vi "PhotonPoseEstimator_lowestAmbiguityStrategy.vi"(10 "CameraResult":T11, 11 "data value reference":T1) -> (1 "Pos Found":bool, 3 "PhotonEstimatedRobotPose":T2={"EstimatedPose"={"Translation3d"={"X"=0.0, "Y"=0.0, "Z"=0.0}, "Rotation3d"={"Q_quaternion"={"R"=1.0, "V"=[0.0, 0.0, 0.0]}}}, "TimeStamp_Seconds"=0.0, "targetsUsed"=[], "Strategy"=enum."LOWEST_AMBIGUITY"} {"targetsUsed"."AltCameraToTarget"."TRANSLATION3D"."Z" format="%14.3f"; "targetsUsed"."AltCameraToTarget"."TRANSLATION3D"."Y" format="%14.3f"; "targetsUsed"."AltCameraToTarget"."TRANSLATION3D"."X" format="%14.3f"; "targetsUsed"."BestCameraToTarget"."TRANSLATION3D"."Z" format="%14.3f"; "targetsUsed"."BestCameraToTarget"."TRANSLATION3D"."Y" format="%14.3f"; "targetsUsed"."BestCameraToTarget"."TRANSLATION3D"."X" format="%14.3f"; "EstimatedPose"."Translation3d"."Z" format="%14.3f"; "EstimatedPose"."Translation3d"."Y" format="%14.3f"; "EstimatedPose"."Translation3d"."X" format="%14.3f"})   [LabVIEW 2019, in "PhotonVisionLib.lvlib"]
doc: "This is an internal function. Use Update or Update_Pipeline instead of this function.\n\nDetermine the best target based the lowest ambiguity."
uses:
  PhotonVisionLib.lvlib
  TypeDef/TargetCornerType.ctl
  <vilib>/Rock Robotics/WPI/ThirdParty/JAS_Junk/TrajLib/TypeDef/TRANSLATION3D.ctl
  <vilib>/Rock Robotics/WPI/ThirdParty/JAS_Junk/TrajLib/Trajectory_Library.lvlib
  <vilib>/Rock Robotics/WPI/ThirdParty/JAS_Junk/TrajLib/TypeDef/QUATERNION.ctl
  <vilib>/Rock Robotics/WPI/ThirdParty/JAS_Junk/TrajLib/TypeDef/ROTATION3D.ctl
  <vilib>/Rock Robotics/WPI/ThirdParty/JAS_Junk/TrajLib/TypeDef/TRANSFORM3D.ctl
  TypeDef/PhotonTrackedTargetType.ctl
  Enum/PhotonPoseStrategy_ENUM.ctl
  <vilib>/Rock Robotics/WPI/ThirdParty/JAS_Junk/TrajLib/TypeDef/POSE3D.ctl
  TypeDef/PhotonEstimatedRobotPoseType.ctl
  TypeDef/PhotonPipelineResultType.ctl
  <vilib>/Rock Robotics/WPI/ThirdParty/JAS_Junk/TrajLib/TypeDef/AprilTag.ctl
  <vilib>/Rock Robotics/WPI/ThirdParty/JAS_Junk/TrajLib/Enum/AprilTagFieldLayoutOrignPosition_ENUM.ctl
  <vilib>/Rock Robotics/WPI/ThirdParty/JAS_Junk/TrajLib/TypeDef/AprilTagFieldLayout.ctl
  TypeDef/PhotonPoseEstimatorType.ctl
  TypeDef/PhotonPNPResultType.ctl
  TypeDef/PhotonMultiTargetPNPResultType.ctl
  TypeDef/PhotonTargetModel.ctl
  Ref/PhotonPipelineResult_REF.ctl
  Ref/PhotonPoseEstimator_REF.ctl
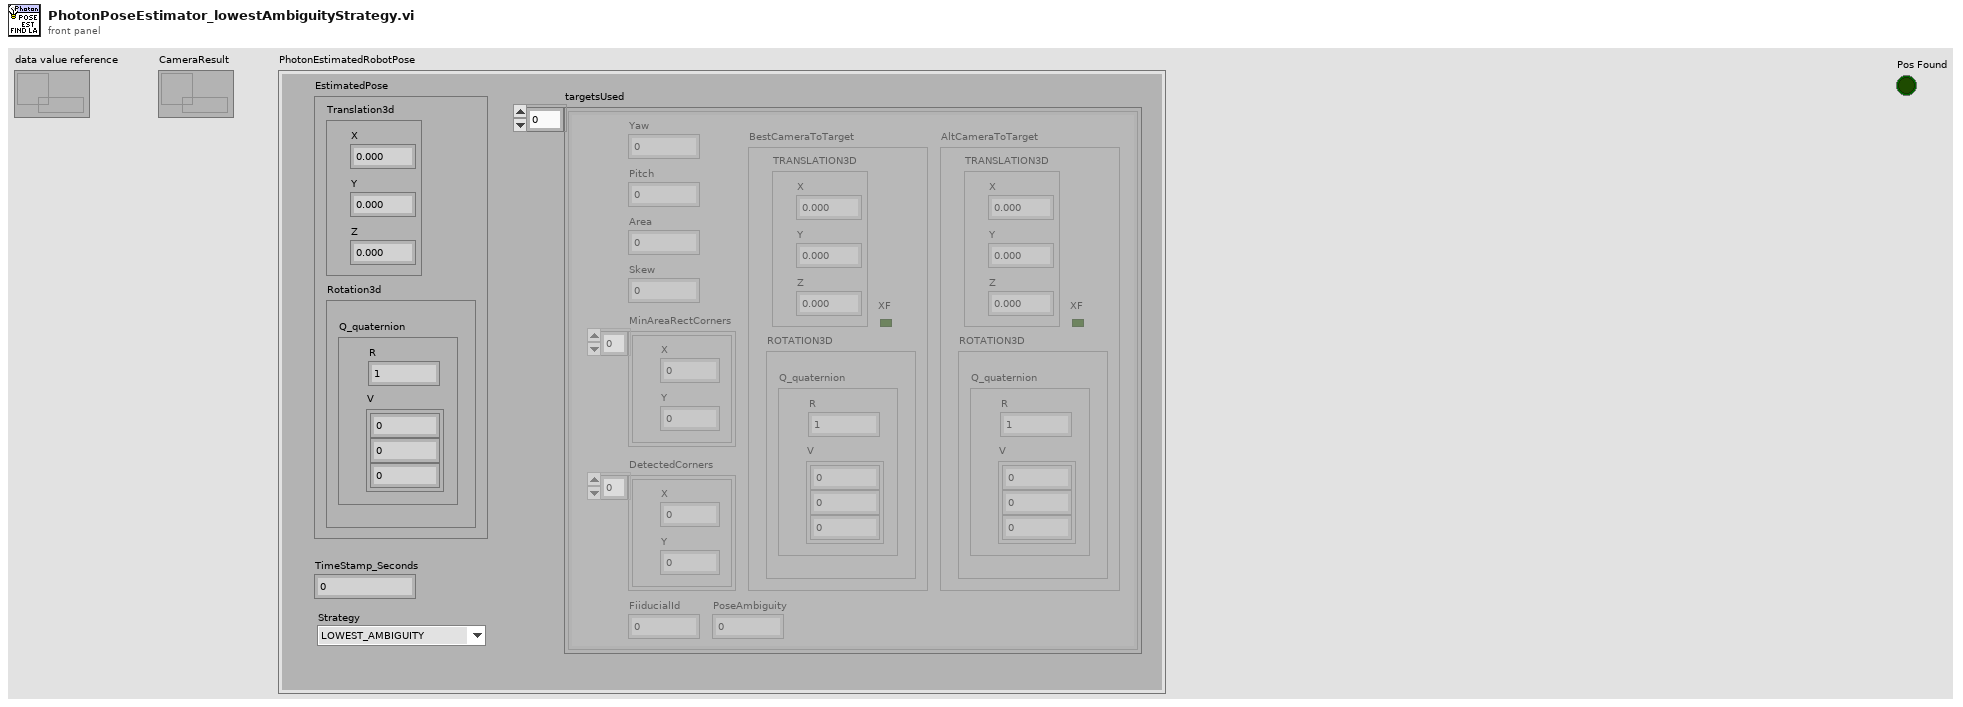
[diagram p1: front panel]
types:
  T1 = typedef "PhotonVisionLib.lvlib/PhotonPoseEstimator_REF.ctl" = refnum<data-value>
  T2 = typedef "PhotonVisionLib.lvlib/PhotonEstimatedRobotPoseType.ctl" = cluster{"EstimatedPose":T3, "TimeStamp_Seconds":dbl, "targetsUsed":T7[], "Strategy":T10}
  T3 = typedef "Trajectory_Library.lvlib/POSE3D.ctl" = cluster{"Translation3d":T4, "Rotation3d":T5}
  T4 = typedef "Trajectory_Library.lvlib/TRANSLATION3D.ctl" = cluster{"X":dbl, "Y":dbl, "Z":dbl}
  T5 = typedef "Trajectory_Library.lvlib/ROTATION3D.ctl" = cluster{"Q_quaternion":T6}
  T6 = typedef "Trajectory_Library.lvlib/QUATERNION.ctl" = cluster{"R":dbl, "V":dbl[]}
  T7 = typedef "PhotonVisionLib.lvlib/PhotonTrackedTargetType.ctl" = cluster{"Yaw":dbl, "Pitch":dbl, "Area":dbl, "Skew":dbl, "MinAreaRectCorners":T8[], "BestCameraToTarget":T9, "FiiducialId":i32, "AltCameraToTarget":T9, "PoseAmbiguity":dbl, "DetectedCorners":T8[]}
  T8 = typedef "PhotonVisionLib.lvlib/TargetCornerType.ctl" = cluster{"X":dbl, "Y":dbl}
  T9 = typedef "Trajectory_Library.lvlib/TRANSFORM3D.ctl" = cluster{"TRANSLATION3D":T4, "ROTATION3D":T5, "XF":bool}
  T10 = typedef "PhotonVisionLib.lvlib/PhotonPoseStrategy_ENUM.ctl" = enum16{"LOWEST_AMBIGUITY", "CLOSEST_TO_CAMERA_HEIGHT", "CLOSEST_TO_REFERENCE_POSE", "CLOSEST_TO_LAST_POSE", "AVERAGE_BEST_TARGETS", "MULTI_TAG_PNP_ON_COPROCESSOR", "MULTI_TAG_PNP_ON_RIO"}
  T11 = typedef "PhotonVisionLib.lvlib/PhotonPipelineResult_REF.ctl" = refnum<data-value>
  T12 = typedef "Trajectory_Library.lvlib/AprilTagFieldLayout.ctl" = cluster{"AprilTagMap":map{i32, T13}, "FieldLength":dbl, "FieldWidth":dbl, "OriginPosition ":T14, "OriginPose3d":T3}
  T13 = typedef "Trajectory_Library.lvlib/AprilTag.ctl" = cluster{"ID":i32, "POSE3D":T3}
  T14 = typedef "Trajectory_Library.lvlib/AprilTagFieldLayoutOrignPosition_ENUM.ctl" = enum16{"kBlueAllianceWallRightSide,", "kRedAllianceWallRightSide,"}
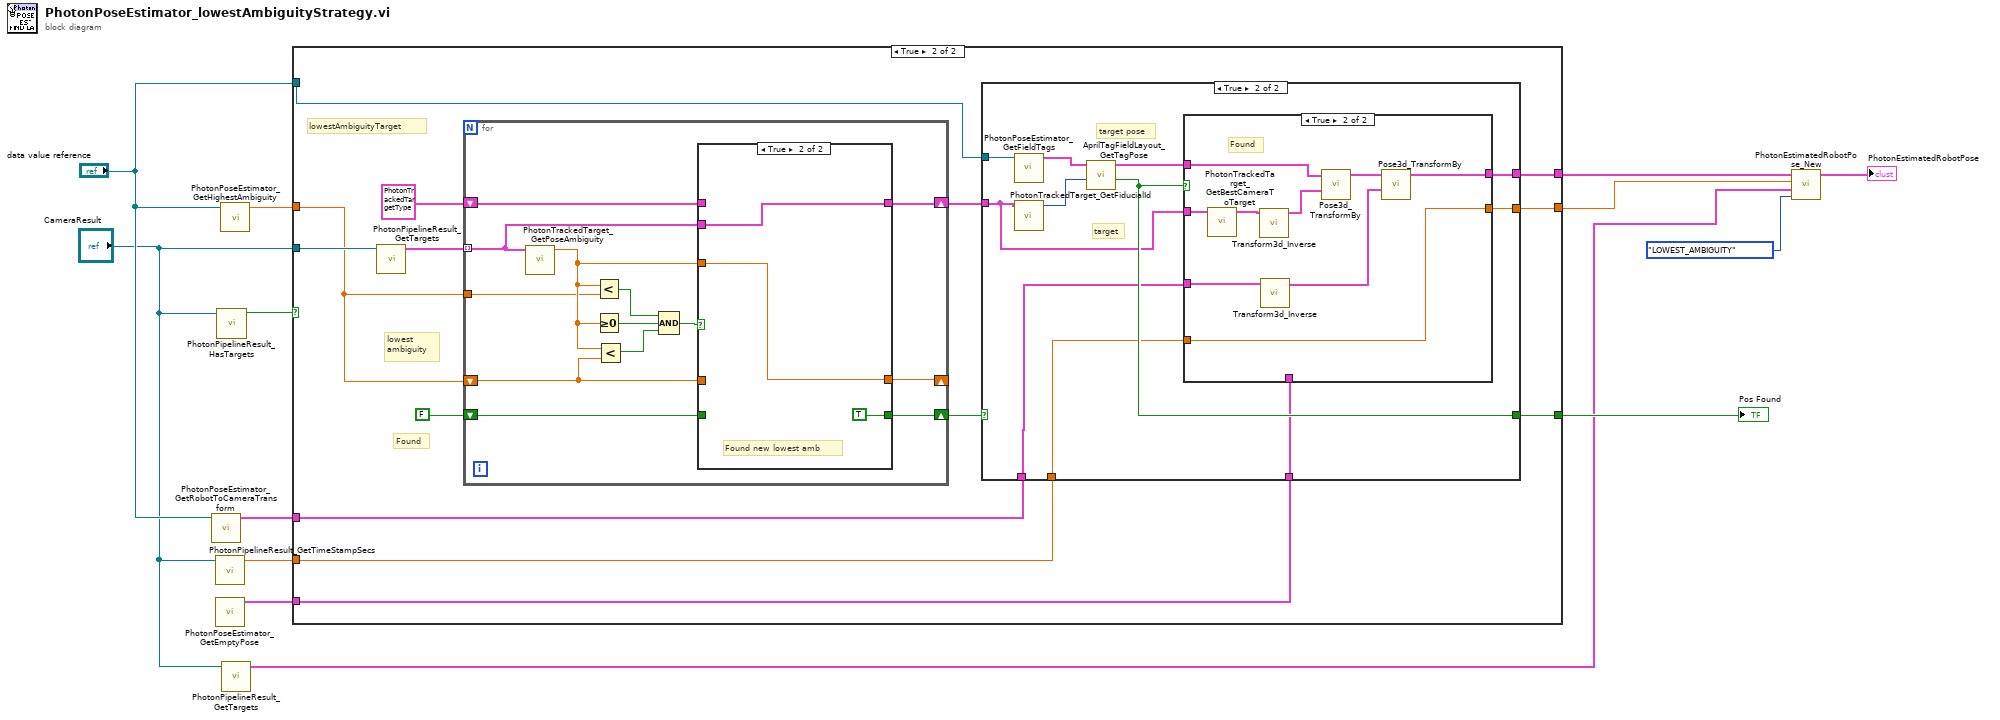
[diagram p0: block diagram]
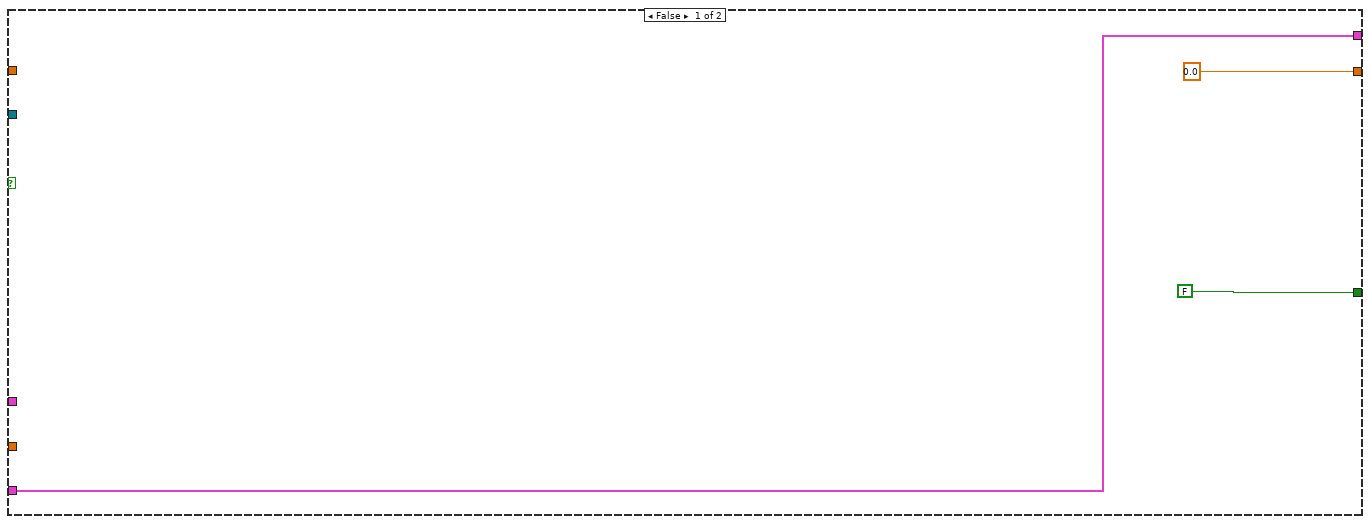
[diagram p2: hidden frame]
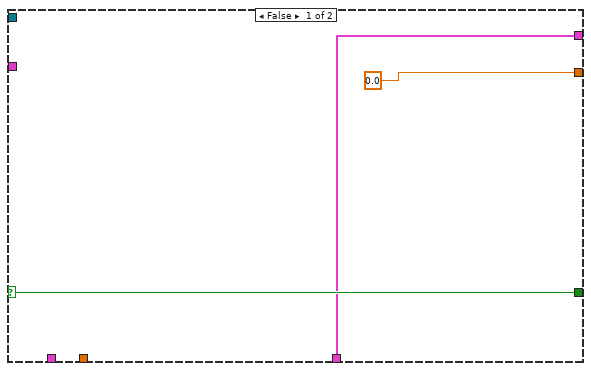
[diagram p3: hidden frame]
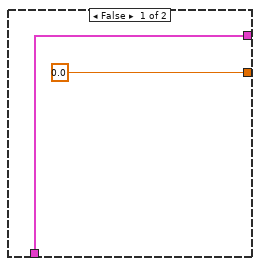
[diagram p4: hidden frame]
diagram:
  n1 = call "PhotonPoseEstimator_GetRobotToCameraTransform.vi"("PhotonPoseEstimator"="data value reference") -> ("RobotToCamera"=w10:T9)  [unwired: 10 in]
  n2 = call "PhotonPipelineResult_GetTimeStampSecs.vi"("PhotonPipelineResult_REF"="CameraResult") -> ("TimeStampSec"=w11:dbl)  [unwired: 10 in]
  n3 = call "PhotonPoseEstimator_GetEmptyPose.vi"() -> ("EmptyPose"=w9:T3)  [unwired: 11 in]
  n4 = call "PhotonPipelineResult_HasTargets.vi"("PhotonPipelineResult_REF"="CameraResult") -> ("HasTargets"=w13:bool)  [unwired: 10 in]
  n5 = call "PhotonPoseEstimator_GetHighestAmbiguity.vi"("PhotonPoseEstimator"="data value reference") -> ("HighestAmbiguity"=w7:dbl)  [unwired: 10 in]
  n6 = call "PhotonPipelineResult_GetTargets.vi"("PhotonPipelineResult_REF"="CameraResult") -> ("Targets"=w1:T7[])  [unwired: 10 in]
  n7 = case shown="True" w13 {
    tunnel: "CameraResult" -> [_ w27]
    tunnel: [FALSE ("Found") w23] -> w12
    tunnel: "data value reference" -> [_ w24]
    tunnel: w11 -> [_ w21]
    tunnel: w10 -> [_ w22]
    tunnel: w9 -> [w15 w20]
    tunnel: w7 -> [_ w17]
    tunnel: [0.0 ("TimeStamp_Seconds") w19] -> w6
    tunnel: [w15 w18] -> w5
    frame False {
    }
    frame True {
      # "lowest\nambiguity"
      # "lowestAmbiguityTarget"
      # "Found"
      n8 = call "PhotonPipelineResult_GetTargets.vi"("PhotonPipelineResult_REF"=w27) -> ("Targets"=w30:T7[])  [unwired: 10 in]
      n9 = for {
        tunnel: w30 -> [w61] mode=indexing
        shift-right: [w60] -> w25
        shift-left: T7 {"Yaw"=0.0, "Pitch"=0.0, "Area"=0.0, "Skew"=0.0, "MinAreaRectCorners"=[], "BestCameraToTarget"={"TRANSLATION3D"={"X"=0.0, "Y"=0.0, "Z"=0.0}, "ROTATION3D"={"Q_quaternion"={"R"=1.0, "V"=[0.0, 0.0, 0.0]}}, "XF"=FALSE}, "FiiducialId"=0, "AltCameraToTarget"={"TRANSLATION3D"={"X"=0.0, "Y"=0.0, "Z"=0.0}, "ROTATION3D"={"Q_quaternion"={"R"=1.0, "V"=[0.0, 0.0, 0.0]}}, "XF"=FALSE}, "PoseAmbiguity"=0.0, "DetectedCorners"=[]} ("PhotonTrackedTarget") -> [w59]
        shift-right: [w65] -> w26
        shift-left: FALSE -> [w62]
        shift-right: [w64] -> _
        shift-left: w17 -> [w63]
        tunnel: w17 -> [w56]
        n10 = call "PhotonTrackedTarget_GetPoseAmbiguity.vi"("TrackedTarget"=w61) -> ("Pose Ambiguity"=w58:dbl)  [unwired: 10 in]
        n11 = Less?(x=w58, y=w56) -> (x < y?=w57:bool)
        n12 = Greater Or Equal To 0?(x=w58) -> (x >= 0?=w68:bool)
        n13 = Less?(x=w58, y=w63) -> (x < y?=w67:bool)
        n14 = Compound Arithmetic op=AND(w57, w68, w67) -> (w66:bool)
        n15 = case shown="True" w66 {
          tunnel: [w70 TRUE] -> w65
          tunnel: [w71 w73] -> w64
          tunnel: w58 -> [_ w73]
          tunnel: w63 -> [w71 _]
          tunnel: w62 -> [w70 _]
          tunnel: w61 -> [_ w72]
          tunnel: [w69 w72] -> w60
          tunnel: w59 -> [w69 _]
          frame False {
          }
          frame True {
            # "Found new lowest amb"
          }
        }
      }
      n16 = case shown="True" w26 {
        selector: w26 -> [w33 _]
        tunnel: w25 -> [_ w38]
        tunnel: w24 -> [_ w44]
        tunnel: [w33 w41] -> w23
        tunnel: w22 -> [_ w40]
        tunnel: w21 -> [_ w37]
        tunnel: w20 -> [w31 w36]
        tunnel: [w31 w35] -> w18
        tunnel: [0.0 ("TimeStamp_Seconds") w34] -> w19
        frame False {
        }
        frame True {
          # "target"
          # "target pose"
          n17 = call "PhotonPoseEstimator_GetFieldTags.vi"("PhotonPoseEstimator"=w44) -> ("AprilTagFieldLayout"=w42:T12)  [unwired: 10 in]
          n18 = call "PhotonTrackedTarget_GetFiducialId.vi"("TrackedTarget"=w38) -> ("Fiducial Id"=w43:i32)  [unwired: 10 in]
          n19 = call <vilib>:"AprilTagFieldLayout_GetTagPose.vi"("TagId"=w43, "AprilTagFieldLayout"=w42) -> ("Found"=w41:bool, "TagPose3d"=w39:T3)  [unwired: 8 in]
          n20 = case shown="True" w41 {
            tunnel: w40 -> [_ w51]
            tunnel: w39 -> [_ w50]
            tunnel: w38 -> [_ w49]
            tunnel: w37 -> [_ w47]
            tunnel: w36 -> [w45 _]
            tunnel: [w45 w48] -> w35
            tunnel: [0.0 ("TimeStamp_Seconds") w47] -> w34
            frame False {
            }
            frame True {
              # "Found"
              n21 = call "PhotonTrackedTarget_GetBestCameraToTarget.vi"("TrackedTarget"=w49) -> ("BestCameraToTarget"=w52:T9)  [unwired: 9 in, 1 out]
              n22 = call <vilib>:"Transform3d_Inverse.vi"("inTransform3d"=w52) -> ("outTransform3d"=w53:T9)  [unwired: 10 in]
              n23 = call <vilib>:"Transform3d_Inverse.vi"("inTransform3d"=w51) -> ("outTransform3d"=w55:T9)  [unwired: 10 in]
              n24 = call <vilib>:"Pose3d_TransformBy.vi"("other Transform3d"=w53, "in Pose3d"=w50) -> ("out POSE3d"=w54:T3)  [unwired: 9 in]
              n25 = call <vilib>:"Pose3d_TransformBy.vi"("other Transform3d"=w55, "in Pose3d"=w54) -> ("out POSE3d"=w48:T3)  [unwired: 9 in]
            }
          }
        }
      }
    }
  }
  "Pos Found" <- w12
  n26 = call "PhotonEstimatedRobotPose_New.vi"("Strategy"=PhotonPoseStrategy_ENUM."LOWEST_AMBIGUITY", "targetsUsed"=w1, "TimeStamp_Seconds"=w6, "EstimatedPose"=w5) -> ("PhotonEstimatedRobotPose"=→"PhotonEstimatedRobotPose":T2)  [unwired: 7 in]
